vi "get_pixel_times.vi"(8 "error in (no error)":errorcluster, 11 "TrajectoryMG100122AODFrameScan in":refnum<class "TrajectoryMG100122AODFrameScan.lvclass">) -> (0 "error out":errorcluster, 1 "AOD equilibration time":dbl[unit], 2 "acquisition time":dbl[unit], 3 "TrajectoryMG100122AODFrameScan out":refnum<class "TrajectoryMG100122AODFrameScan.lvclass">, 4 "total pixel time":dbl[unit])   [LabVIEW 2010, in "TrajectoryMG100122AODFrameScan.lvclass"]
uses:
  TrajectoryMG100122AODFrameScan.lvclass
  FPGAWrapper/FPGAWrapperMH120124AOD/FPGAWrapperMH120124FrameScan_PXI7813R/FPGAWrapperMH120124FrameScan_PXI7813R.lvclass
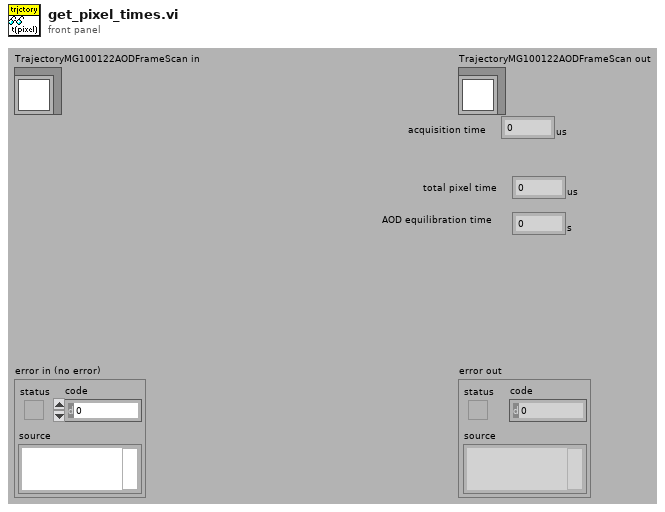
[diagram p1: front panel]
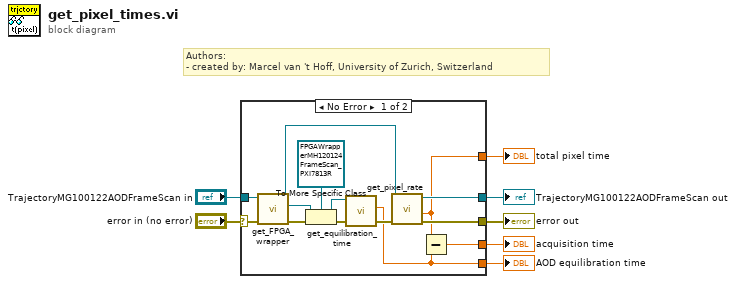
[diagram p0: block diagram]
diagram:
  # "Authors: \n- created by: Marcel van 't Hoff, University of Zurich, Switzerland"
  n1 = case shown="No Error" "error in (no error)" {
    selector: "error in (no error)" -> [w17 w22]
    tunnel: [w21 w22] -> w6
    tunnel: [w20 w23] -> w4
    tunnel: "TrajectoryMG100122AODFrameScan in" -> [w19 w23]
    tunnel: [w10 _] -> w3
    tunnel: [w9 _] -> w2
    tunnel: [w8 _] -> w1
    frame No Error {
      n2 = call-dynamic "get_FPGA_wrapper.vi"("error in (no error)"=w17, "TrajectoryMG100122GenericFPGA in"=w19) -> ("error out"=w16:errorcluster, "GenericFPGAWrapper.lvclass"=w14:refnum<class "GenericFPGAWrapper.lvclass">, "TrajectoryMG100122GenericFPGA out"=w18:refnum<class "TrajectoryMG100122AODFrameScan.lvclass">)  [unwired: 7 in]
      n3 = To More Specific Class(target class=refnum<class "FPGAWrapperMH120124FrameScan_PXI7813R.lvclass"> refnum ("FPGAWrapperMH120124FrameScan_PXI7813R.lvclass"), reference=w14, error in=w16) -> (specific class reference=w13:refnum<class "FPGAWrapperMH120124FrameScan_PXI7813R.lvclass">, error out=w12:errorcluster)
      n4 = call-dynamic "get_equilibration_time.vi"("error in (no error)"=w12, "FPGAWrapperMH120124FrameScan_PXI7813R in"=w13) -> ("error out"=w11:errorcluster, "AOD equilibration time"=w9:dbl[unit])  [unwired: 7 in, 1 out]
      n5 = call-dynamic "get_pixel_rate.vi"("error in (no error)"=w11, "GenericTrajectory in"=w18) -> ("error out"=w21:errorcluster, "pixel dwell time"=w10:dbl[unit], "GenericTrajectory out"=w20:refnum<class "TrajectoryMG100122AODFrameScan.lvclass">)  [unwired: 6 in, 1 out]
      n6 = Subtract(x=w10, y=w9) -> (x-y=w8:dbl[unit])
    }
    frame Error {
    }
  }
  "error out" <- w6
  "TrajectoryMG100122AODFrameScan out" <- w4
  "total pixel time" <- w3
  "AOD equilibration time" <- w2
  "acquisition time" <- w1
